vi "Ejercicio1_Sumadora Sencilla.vi"() -> ()   [LabVIEW 2018]
panel:
  in  "stop":bool
  out "Suma":dbl
  in  "Número 2":dbl
  in  "Número 1":dbl
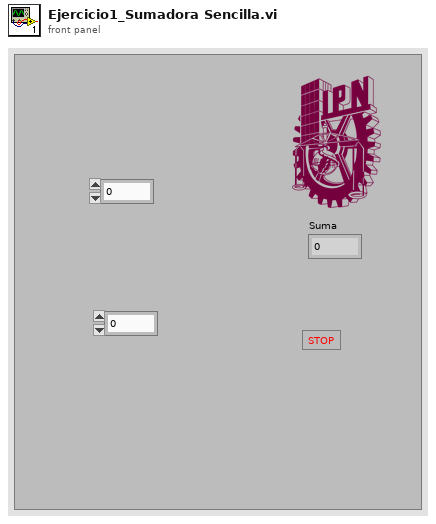
[diagram p1: front panel]
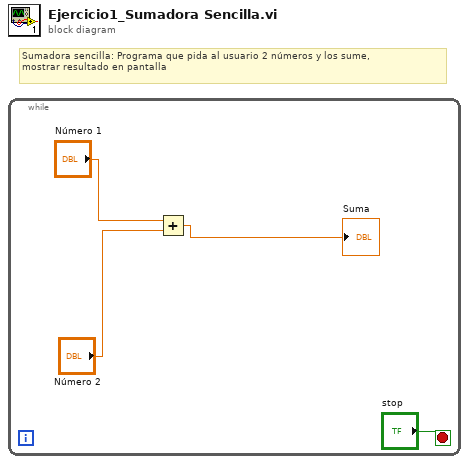
[diagram p0: block diagram]
diagram:
  # "Sumadora sencilla: Programa que pida al usuario 2 números y los sume,\nmostrar resultado en pantalla"
  n1 = while {
    stop <- "stop" stop-if-true
    n2 = Add(x="Número 1", y="Número 2") -> (x+y=→"Suma":dbl)
  }
